vi "receive.vi"(8 "error in (no error)":errorcluster, 11 "TCP_IP.lvclass":refnum<class "TCP_IP.lvclass">) -> (0 "error out":errorcluster, 2 "data out":string)   [LabVIEW 2013, in "TCP_IP.lvclass"]
uses:
  TCP_IP.lvclass
  TCP_IP.lvclass/TCP_IP.ctl
  Experiment/Globals.vi
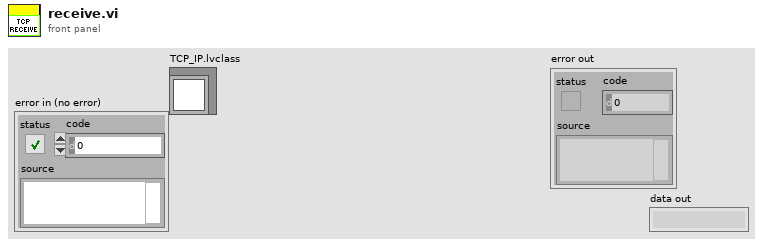
[diagram p1: front panel]
types:
  T1 = enum16{"Standard", "Buffered", "CRLF", "Immediate"}
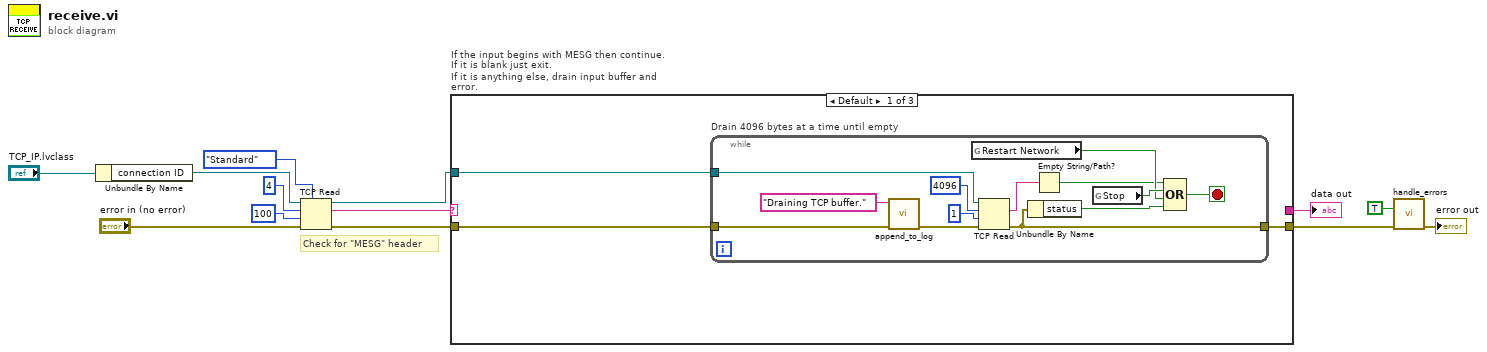
[diagram p0: block diagram]
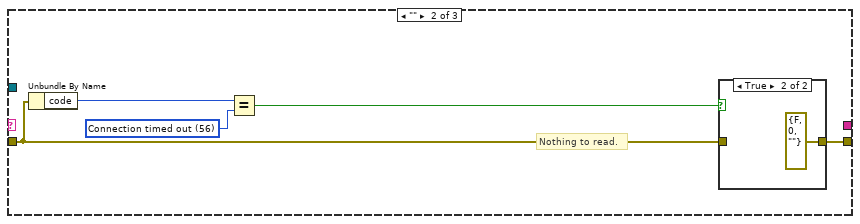
[diagram p2: hidden frame]
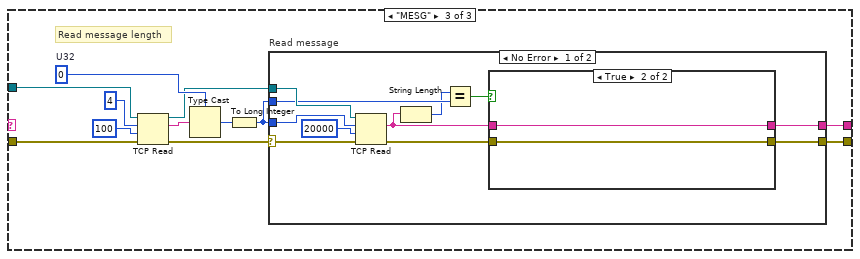
[diagram p4: hidden frame]
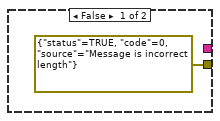
[diagram p5: hidden frame]
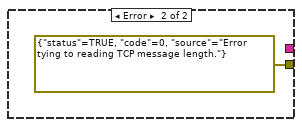
[diagram p6: hidden frame]
diagram:
  # "Check for \"MESG\" header"
  n1 = Unbundle By Name("TCP_IP.lvclass") -> ("connection ID"=w4:refnum<k5>)
  n2 = TCP Read(connection ID=w4, bytes to read=4, error in (no error)="error in (no error)", 7:T1."Standard" ("mode (standard)"), 9:100 ("timeout ms (25000)")) -> (connection ID out=w8:refnum<k5>, data out=w6:string, error out=w9:errorcluster)
  n3 = case "If the input begins with MESG then continue.\nIf it is blank just exit.\nIf it is anything else, drain input buffer and error." shown="Default" w6 {
    tunnel: w9 -> [w14 w30 w48]
    tunnel: w8 -> [w16 _ w46]
    tunnel: [w15 w31 w39] -> w7
    tunnel: [_ _ w38] -> w5
    frame Default {
      n4 = while "Drain 4096 bytes at a time until empty" {
        tunnel: w16 -> [w28]
        tunnel: [w17] -> w15
        tunnel: w14 -> [w25]
        stop <- w19 stop-if-true
        n5 = call "append_to_log.vi"("error in"=w25, "string"="Draining TCP buffer.") -> ("error out"=w24:errorcluster)  [unwired: 9 in]
        n6 = global read "Globals.vi" "Restart Network"() -> (w21:bool)
        n7 = TCP Read(connection ID=w28, bytes to read=4096, error in (no error)=w24, 9:1 ("timeout ms (25000)")) -> (data out=w27:string, error out=w17:errorcluster)  [unwired: 1 in, 1 out]
        n8 = Unbundle By Name(w17) -> ("status"=w18:bool)
        n9 = Empty String/Path?(string/path=w27) -> (empty?=w20:bool)
        n10 = global read "Globals.vi" "Stop"() -> (w22:bool)
        n11 = Compound Arithmetic op=OR(w20, w22, w21, w18) -> (w19:bool)
      }
    }
    frame "" {
      w34 = 56 items=["No Error", "Argument Error", "Memory Full", "Out of Zone", "End of File", "File Already Open", "Generic File IO Error", "File Not Found", "File Permission Error", "Disk Full", "Duplicate Path", "Too Many Files Open", "Not Enabled", "Resource File Not Found", "Cannot Add Resource", "Resource Not Found", "Image Not Found", "Image Memory Error", "Pen Does Not Exist", "Config Bad Type", "Config Token Not Found", "Config Parse Error", "Config Memory Error", "Bad External Code Format", "Bad External Code Offset", "External Code Not Present", "Null Window", "Destroy Window Mixup", "Null Menu", "Print Aborted", "Bad Print Record", "Print Driver Error", "Windows Error During Print", "Memory Error During Print", "Print Dialog Error", "Generic Print Error", "Invalid Device Refnum", "Device Not Found", "Device Parameter Error", "Device Unit Error", "Can't Open Device", "Device Call Aborted", "Generic Error", "Cancelled By User", "Object ID Too Low", "Object ID Too High", "Object Not In Heap", "Unknown Heap", "Bad DefProc ID", "DefProc Not In Table", "Message Out Of Range", "Null Method", "Unknown Message", "Manager Call Not Supported", "Bad address", "Connection In progress", "Connection timed out", "Connection is already in progress", "Network attribute not supported", "Network error", "Address in use", "System out of memory", "Connection aborted", "Connection refused", "Connection is not connected", "Connection is already connected", "Connection closed", "Initialize error (interapplication manager)", "Bad occurrence", "Wait on unbound occurrence handler", "Occurrence queue overflow", "Bad path", "Semaphore not signaled", "Unrecognized type (interapplication manager)"] ("1st Error to Convert")
      # "Nothing to read."
      n12 = Unbundle By Name(w30) -> ("code"=w33:i32)
      n13 = Equal?(x=w33, y=w34) -> (x = y?=w32:bool)
      n14 = case shown="True" w32 {
        tunnel: [w35 errorcluster {"status"=FALSE, "code"=0, "source"=""} ("error constant")] -> w31
        tunnel: w30 -> [w35 _]
        frame False {
        }
        frame True {
        }
      }
    }
    frame "MESG" {
      w42 = u32 0  # U32
      # "Read message length"
      n15 = TCP Read(connection ID=w46, bytes to read=4, error in (no error)=w48, 9:100 ("timeout ms (25000)")) -> (connection ID out=w40:refnum<k5>, data out=w43:string, error out=w44:errorcluster)  [unwired: 1 in]
      n16 = Type Cast(type=w42, x=w43) -> (*(type *) &x=w41:u32)
      n17 = To Long Integer(number=w41) -> (32bit integer=w37:i32)
      n18 = case "Read message" shown="No Error" w44 {
        selector: w44 -> [w58 _]
        tunnel: w37 -> [w59 _]
        tunnel: w40 -> [w57 _]
        tunnel: [w51 errorcluster {"status"=TRUE, "code"=0, "source"="Error tying to reading TCP message length."} ("error constant")] -> w39
        tunnel: [w52 _] -> w38
        tunnel: w37 -> [w56 _]
        frame No Error {
          n19 = TCP Read(connection ID=w57, bytes to read=w59, error in (no error)=w58, 9:20000 ("timeout ms (25000)")) -> (data out=w53:string, error out=w50:errorcluster)  [unwired: 1 in, 1 out]
          n20 = String Length(string=w53) -> (length=w55:i32)
          n21 = Equal?(x=w55, y=w56) -> (x = y?=w54:bool)
          n22 = case shown="True" w54 {
            tunnel: w53 -> [_ w62]
            tunnel: [_ w62] -> w52
            tunnel: [errorcluster {"status"=TRUE, "code"=0, "source"="Message is incorrect length"} ("error constant") w61] -> w51
            tunnel: w50 -> [_ w61]
            frame False {
            }
            frame True {
            }
          }
        }
        frame Error {
        }
      }
    }
  }
  "data out" <- w5
  n23 = call "handle_errors.vi"("Restart Network"=TRUE, "error in (no error)"=w7) -> ("error out"=→"error out":errorcluster)  [unwired: 13 in]
